vi "430_TCP_Query.vi"(8 "error in (no error)":errorcluster, 9 "Timeout":i32=1000, 10 "Command":string, 11 "connection ID":refnum<k5>) -> (0 "error out":errorcluster, 1 "Bytes Read":i32, 2 "Response":string, 3 "connection ID out":refnum<k5>, 4 "Bytes Written":i32)   [LabVIEW 2017]
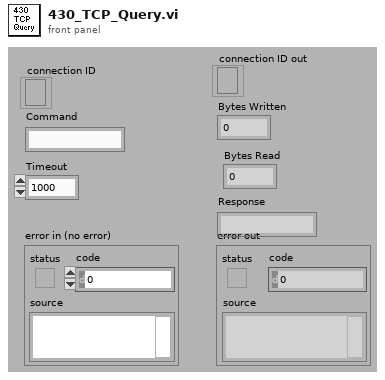
[diagram p1: front panel]
types:
  T1 = enum16{"Standard", "Buffered", "CRLF", "Immediate"}
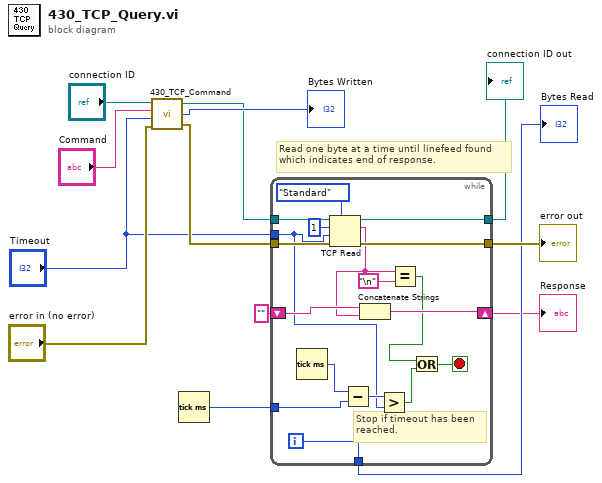
[diagram p0: block diagram]
diagram:
  # "Read one byte at a time until linefeed found\nwhich indicates end of response."
  n1 = call "430_TCP_Command.vi"("error in (no error)"="error in (no error)", "Timeout"="Timeout", "Command"="Command", "connection ID"="connection ID") -> ("error out"=w7:errorcluster, "bytes written"=→"Bytes Written":i32, "connection ID out"=w9:refnum<k5>)
  n2 = Tick Count (ms)() -> (millisecond timer value=w1:u32)
  n3 = while {
    tunnel: w9 -> [w31]
    tunnel: [w30] -> w8
    tunnel: w7 -> [w29]
    tunnel: [w28] -> w6
    tunnel: [w27] -> w5
    shift-right: [w21] -> w2
    shift-left: "" -> [w23]
    tunnel: "Timeout" -> [w14]
    tunnel: w1 -> [w19]
    i -> [w27]
    stop <- w15 stop-if-true
    # "Stop if timeout has been\nreached."
    n4 = Tick Count (ms)() -> (millisecond timer value=w20:u32)
    n5 = TCP Read(connection ID=w31, bytes to read=1, error in (no error)=w29, 7:T1."Standard" ("mode (standard)"), 9:w14) -> (connection ID out=w30:refnum<k5>, data out=w22:string, error out=w28:errorcluster)
    n6 = Subtract(x=w20, y=w19) -> (x-y=w18:u32)
    n7 = Concatenate Strings(w23, w22) -> (w21:string)
    n8 = Greater?(x=w18, y=w14) -> (0:w17:bool)
    n9 = Equal?(x=w22, y="\n") -> (x = y?=w16:bool)
    n10 = Or(x=w16, y=w17) -> (x .or. y?=w15:bool)
  }
  "error out" <- w6
  "Bytes Read" <- w5
  "Response" <- w2
  "connection ID out" <- w8
